vi "EvaluateDataFlowBlock.vi"(8 "error in (no error)":errorcluster, 9 "data":T2, 10 "config":T1, 11 "Qbus":refnum<class "Qbus.lvclass">) -> (0 "error out":errorcluster, 2 "config out":T1)   [LabVIEW 2017, in "EmsaDataEventCreator.lvlib"]
uses:
  <vilib>/addons/InsightCM/Devices/Shared/Emsa/EmsaDataEventCreator/EmsaDataEventCreator.lvlib
  <vilib>/addons/InsightCM/Devices/Shared/Common/DataFlow/controls/Data.ctl
  <vilib>/addons/InsightCM/Utilities/DataAccessors/controls/wfmSGL_DVR.ctl
  <vilib>/addons/PointValueMap/controls/PointMap.ctl
  <vilib>/addons/InsightCM/Devices/Shared/Common/DataFlow/controls/Type.ctl
  <vilib>/addons/Qbus/Qbus.lvclass
  <vilib>/addons/InsightCM/Devices/Shared/Emsa/EmsaDataEventCreator/controls/config.ctl
  <vilib>/addons/InsightCM/Devices/Shared/Emsa/EmsaDataEventCreator/controls/DataEventConfig.ctl
  <vilib>/addons/InsightCM/Devices/Shared/Emsa/EmsaDataEventCreator/controls/SweepParams.ctl
  <vilib>/addons/InsightCM/Devices/Shared/Common/DataEventCreator/controls/Reason.ctl
  <vilib>/addons/PointValueMap/subVIs/Point_Read_string.vi
  <vilib>/addons/PointValueMap/PointValueMap.lvlib
  <vilib>/addons/InsightCM/Devices/Shared/Common/DataEventCreator/DataEventCreator.lvlib
  <vilib>/addons/InsightCM/Devices/Shared/Common/DataFlow/DataFlow.lvlib
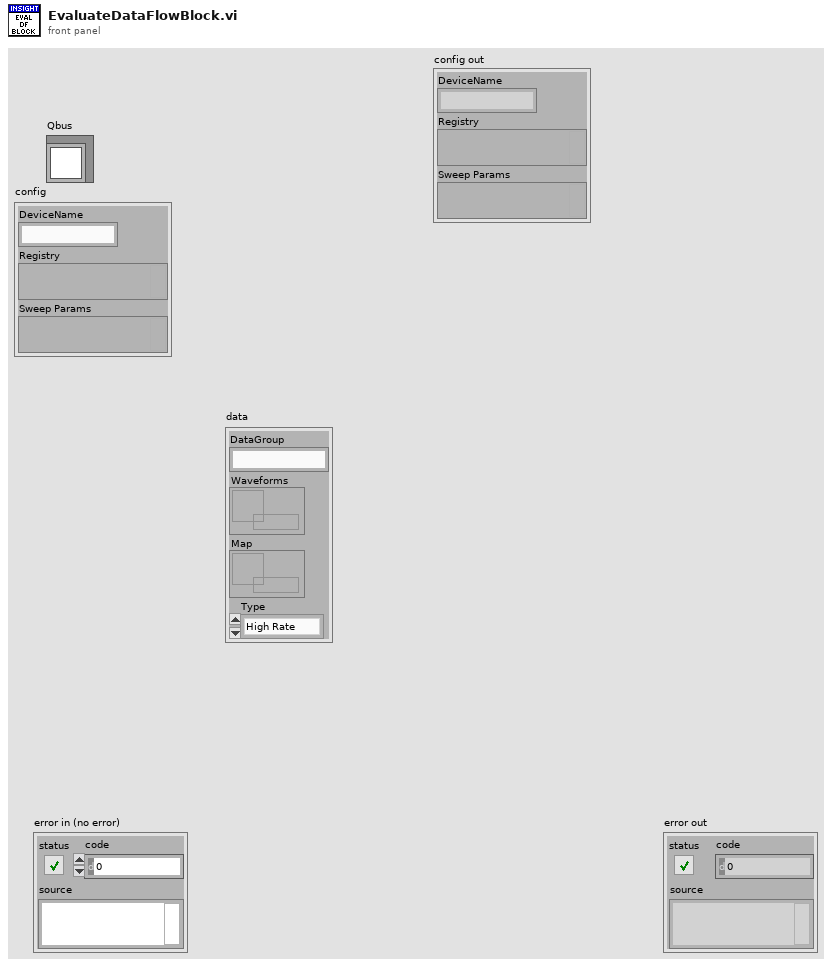
[diagram p1: front panel]
types:
  T1 = typedef "EmsaDataEventCreator.lvlib/config.ctl" = cluster{"DeviceName":string, "Registry":variant, "Sweep Params":variant}
  T2 = typedef "DataFlow.lvlib/Data.ctl" = cluster{"DataGroup":string, "Waveforms":T3, "Map":T4, "Type":T5}
  T3 = typedef "wfmSGL_DVR.ctl" = refnum<data-value>
  T4 = typedef "PointValueMap.lvlib/PointMap.ctl" = refnum<data-value>
  T5 = typedef "DataFlow.lvlib/Type.ctl" = enum16{"High Rate", "Low Rate", "Burst Mode"}
  T6 = typedef "EmsaDataEventCreator.lvlib/SweepParams.ctl" = cluster{"CollectOnEnter":bool, "CollectOnExit":bool}
  T7 = typedef "DataEventCreator.lvlib/Reason.ctl" = enum16{"Periodic Event", "Delta EU Event", "Trend Event", "Alarm Event", "User Event", "Enter Operating State", "Exit Operating State", "Multiple Events", "Other"}
  T8 = typedef "EmsaDataEventCreator.lvlib/DataEventConfig.ctl" = cluster{"OpState":string, "ExitOpState":bool, "Reason":string, "StreamId":string, "Map":T4, "DataSetIds":variant, "IncludeWaveforms":bool, "TrendPointsOnly":bool, "Sweep Params":T6}
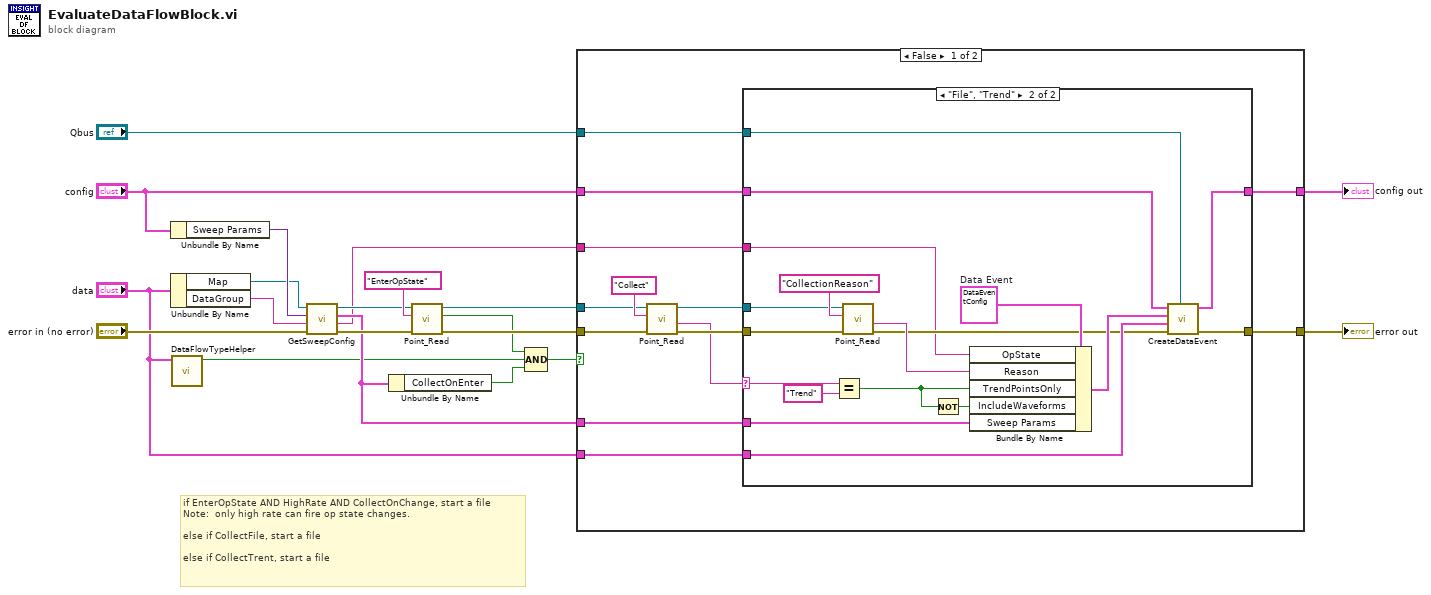
[diagram p0: block diagram]
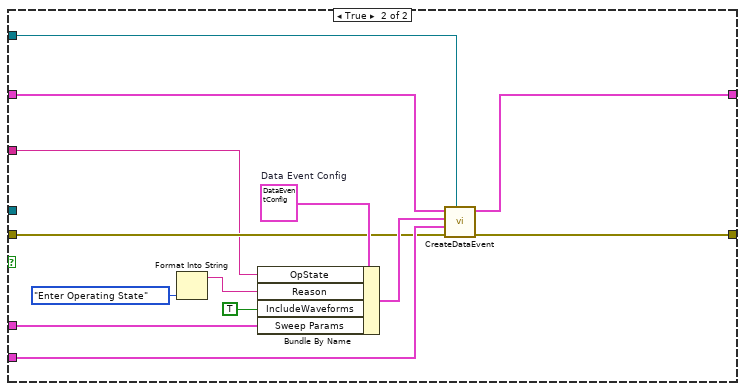
[diagram p3: hidden frame]
diagram:
  # "if EnterOpState AND HighRate AND CollectOnChange, start a file\nNote:  only high rate can fire op state changes.\n\nelse if CollectFile, start a file\n\nelse if CollectTrent, start a file"
  n1 = Unbundle By Name("config") -> ("Sweep Params"=w10:variant)
  n2 = Unbundle By Name("data") -> ("Map"=w3:T4, "DataGroup"=w9:string)
  n3 = call <vilib>:"DataFlowTypeHelper.vi"("data"="data") -> ("high rate"=w1:bool)  [unwired: 8 in, 2 out]
  n4 = call <vilib>:"GetSweepConfig.vi"("error in (no error)"="error in (no error)", "DataGroup"=w9, "AcqParams"=w10, "map in"=w3) -> ("error out"=w15:errorcluster, "OpState"=w11:string, "sweep config"=w12:T6, "map out"=w13:T4)  [unwired: 4 in]
  n5 = Unbundle By Name(w12) -> ("CollectOnEnter"=w6:bool)
  n6 = call-poly <vilib>:"Point_Read.vi"("Error In"=w15, "Tag"="EnterOpState", "Map"=w13) -> ("Error Out"=w18:errorcluster, "Found?"=w4:bool, "Map Out"=w16:T4)  [unwired: 3 in, 3 out]
  n7 = Compound Arithmetic op=AND(w4, w1, w6) -> (w5:bool)
  n8 = case shown="False" w5 {
    tunnel: [w32 w65] -> w19
    tunnel: "config" -> [w25 w55]
    tunnel: [w22 w62] -> w8
    tunnel: w12 -> [w26 w54]
    tunnel: w11 -> [w27 w56]
    tunnel: w18 -> [w30 w57]
    tunnel: "data" -> [w23 w64]
    tunnel: "Qbus" -> [w24 w61]
    tunnel: w16 -> [w31 _]
    frame False {
      n9 = call-poly <vilib>:"Point_Read.vi"("Error In"=w30, "Tag"="Collect", "Map"=w31) -> ("Error Out"=w28:errorcluster, "Value"=w21:string, "Map Out"=w29:T4)  [unwired: 3 in, 3 out]
      n10 = case shown="\"File\", \"Trend\"" w21 {
        selector: w21 -> [_ w38]
        tunnel: w29 -> [_ w46]
        tunnel: w28 -> [w34 w47]
        tunnel: [w34 w51] -> w32
        tunnel: w27 -> [_ w40]
        tunnel: w26 -> [_ w41]
        tunnel: w25 -> [w35 w43]
        tunnel: w24 -> [_ w49]
        tunnel: w23 -> [_ w52]
        tunnel: [w35 w50] -> w22
        frame Default {
        }
        frame "File", "Trend" {
          w44 = T8 {"OpState"="", "ExitOpState"=FALSE, "Reason"="", "StreamId"="", "Map"=refnum, "DataSetIds"=variant, "IncludeWaveforms"=FALSE, "TrendPointsOnly"=FALSE, "Sweep Params"={"CollectOnEnter"=FALSE, "CollectOnExit"=FALSE}}  # Data Event
          n11 = Equal?(x=w38, y="Trend") -> (x = y?=w36:bool)
          n12 = call-poly <vilib>:"Point_Read.vi"("Error In"=w47, "Tag"="CollectionReason", "Map"=w46) -> ("Error Out"=w42:errorcluster, "Value"=w45:string)  [unwired: 3 in, 4 out]
          n13 = Not(x=w36) -> (.not. x?=w37:bool)
          n14 = Bundle By Name(cluster=w44, "OpState"=w40, "Reason"=w45, "TrendPointsOnly"=w36, "IncludeWaveforms"=w37, "Sweep Params"=w41) -> (w53:T8)
          n15 = call <vilib>:"CreateDataEvent.vi"("Qbus"=w49, "error in (no error)"=w42, "data flow"=w52, "data event config"=w53, "config"=w43) -> ("error out"=w51:errorcluster, "config out"=w50:T1)  [unwired: 5 in]
        }
      }
    }
    frame True {
      w58 = T8 {"OpState"="", "ExitOpState"=FALSE, "Reason"="", "StreamId"="", "Map"=refnum, "DataSetIds"=variant, "IncludeWaveforms"=FALSE, "TrendPointsOnly"=FALSE, "Sweep Params"={"CollectOnEnter"=FALSE, "CollectOnExit"=FALSE}}  # Data Event Config
      n16 = Format Into String(Reason."Enter Operating State" ("Reason")) -> (resulting string=w66:string)  [unwired: 3 in, 1 out]
      n17 = Bundle By Name(cluster=w58, "OpState"=w56, "Reason"=w66, "IncludeWaveforms"=TRUE, "Sweep Params"=w54) -> (w63:T8)
      n18 = call <vilib>:"CreateDataEvent.vi"("Qbus"=w61, "error in (no error)"=w57, "data flow"=w64, "data event config"=w63, "config"=w55) -> ("error out"=w65:errorcluster, "config out"=w62:T1)  [unwired: 5 in]
    }
  }
  "error out" <- w19
  "config out" <- w8
